vi "test_angle_gps-xy-domain.vi"() -> ()   [LabVIEW 2018]
uses:
  <vilib>/Utility/miscctls.llb/LVPointDoubleTypeDef.ctl
panel:
  out "추가된 배열":T1[](array[typedef])
  out "deg_gps-base":dbl format="%.1f"
  out "slope":dbl format="%.1f"
  out "XY graph":cluster{"X":dbl, "Y":dbl}[](graph)
  in  "정지":bool
  in  "point n+1":T1 {"X" format="%.2f"; "Y" format="%.2f"}
  in  "point n":T1 {"X" format="%.2f"; "Y" format="%.2f"}
  in  "dt":u32=10
  out "XY 그래프":cluster{"X":dbl, "Y":dbl}[](graph)
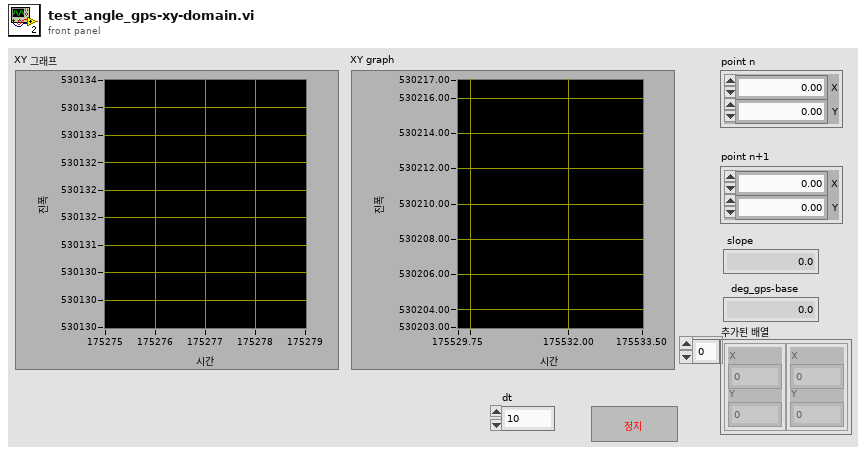
[diagram p1: front panel]
types:
  T1 = typedef "LVPointDoubleTypeDef.ctl" = cluster{"X":dbl, "Y":dbl}
  T2 = cluster{"position":cluster{"X":dbl, "Y":dbl}, "heading":dbl}[]
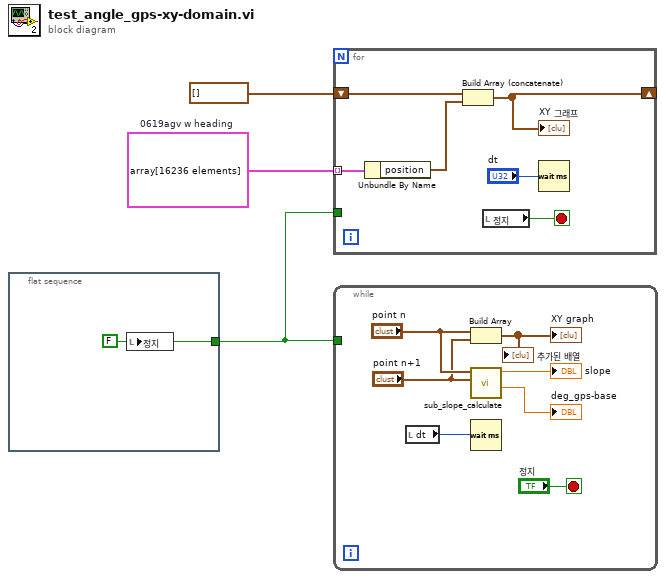
[diagram p0: block diagram]
diagram:
  w3 = T2 array[16236 elements]  # 0619agv w heading
  n1 = flat-sequence {
    tunnel: [w4] -> w1
    frame #0 {
      w4 = FALSE ("정지")
      n2 = local write "정지"(w4) -> ()
    }
  }
  n3 = for {
    tunnel: w3 -> [w10] mode=indexing
    shift-right: [w7] -> _
    shift-left: cluster{"X":dbl, "Y":dbl}[] [] -> [w9]
    tunnel: w1 -> [_]
    stop <- w5 stop-if-true
    n4 = Unbundle By Name(w10) -> ("position"=w8:cluster{"X":dbl, "Y":dbl})
    n5 = Build Array (concatenate)(w9, w8) -> (w7:cluster{"X":dbl, "Y":dbl}[])
    "XY 그래프" <- w7
    n6 = local read "정지"() -> (w5:bool)
    n7 = Wait (ms)(milliseconds to wait="dt") -> ()  [unwired: 1 out]
  }
  n8 = while {
    tunnel: w1 -> [_]
    stop <- "정지" stop-if-true
    n9 = local read "dt"() -> (w17:u32)
    n10 = Build Array("point n", "point n+1") -> (→"XY graph" →"추가된 배열":T1[])
    n11 = call "sub_slope_calculate.vi"("point n+1"="point n+1", "point n"="point n") -> ("deg_gps-base"=→"deg_gps-base":dbl, "slope"=→"slope":dbl)  [unwired: 7 in, 1 out]
    n12 = Wait (ms)(milliseconds to wait=w17) -> ()  [unwired: 1 out]
  }
